vi "calculateDateFormate.vi"(8 "Error In":errorcluster, 11 "Shift":string) -> (0 "Error Out":errorcluster, 2 "Special Date Formate":string, 3 "Production Date":string)   [LabVIEW 2018]
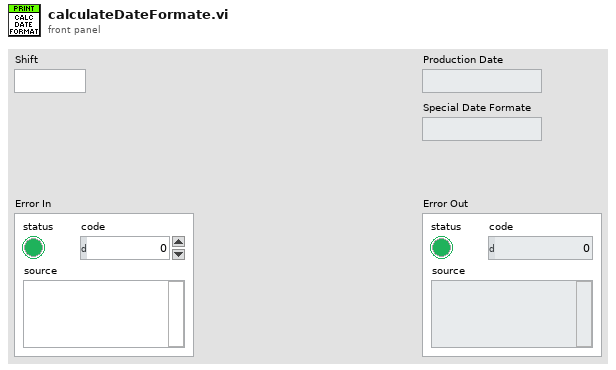
[diagram p1: front panel]
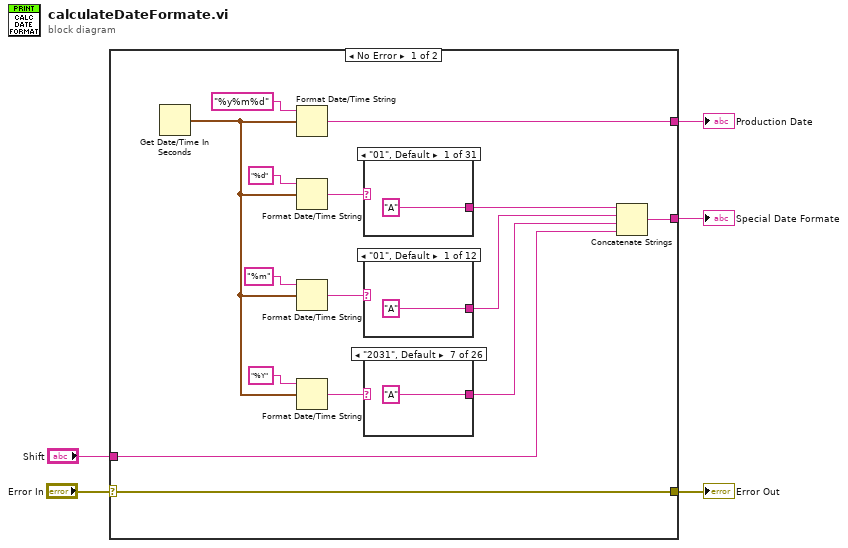
[diagram p0: block diagram]
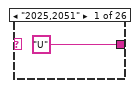
[diagram p2: hidden frame]
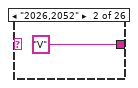
[diagram p3: hidden frame]
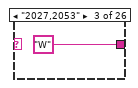
[diagram p4: hidden frame]
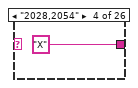
[diagram p5: hidden frame]
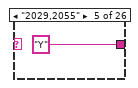
[diagram p6: hidden frame]
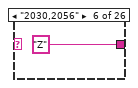
[diagram p7: hidden frame]
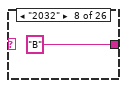
[diagram p8: hidden frame]
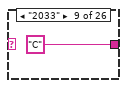
[diagram p9: hidden frame]
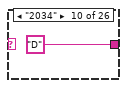
[diagram p10: hidden frame]
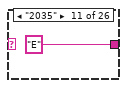
[diagram p11: hidden frame]
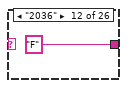
[diagram p12: hidden frame]
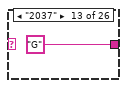
[diagram p13: hidden frame]
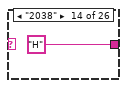
[diagram p14: hidden frame]
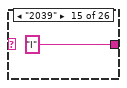
[diagram p15: hidden frame]
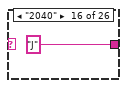
[diagram p16: hidden frame]
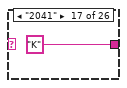
[diagram p17: hidden frame]
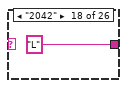
[diagram p18: hidden frame]
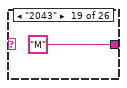
[diagram p19: hidden frame]
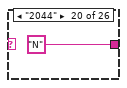
[diagram p20: hidden frame]
diagram:
  n1 = case shown="No Error" "Error In" {
    selector: "Error In" -> [w20 w90]
    tunnel: [w20 w90] -> w4
    tunnel: "Shift" -> [w10 _]
    tunnel: [w9 _] -> w2
    tunnel: [w6 _] -> w1
    frame No Error {
      n2 = Get Date/Time In Seconds() -> (seconds since 1Jan1904=w7:timestamp)
      n3 = Format Date/Time String(time format string (%c)="%y%m%d", seconds (now)=w7) -> (date/time string=w6:string)  [unwired: 1 in]
      n4 = Format Date/Time String(time format string (%c)="%d", seconds (now)=w7) -> (date/time string=w17:string)  [unwired: 1 in]
      n5 = Format Date/Time String(time format string (%c)="%m", seconds (now)=w7) -> (date/time string=w18:string)  [unwired: 1 in]
      n6 = Format Date/Time String(time format string (%c)="%Y", seconds (now)=w7) -> (date/time string=w19:string)  [unwired: 1 in]
      n7 = case shown="\"01\", Default" w17 {
        tunnel: ["A" "B" "C" "D" "E" "F" "G" "H" "I" "J" "K" "L" "M" "N" "O" "P" "Q" "R" "S" "T" "U" "V" "W" "X" "Y" "Z" "1" "2" "3" "4" "5"] -> w13
        frame "01", Default {
        }
        frame "02" {
        }
        frame "03" {
        }
        frame "04" {
        }
        frame "05" {
        }
        frame "06" {
        }
        frame "07" {
        }
        frame "08" {
        }
        frame "09" {
        }
        frame "10" {
        }
        frame "11" {
        }
        frame "12" {
        }
        frame "13" {
        }
        frame "14" {
        }
        frame "15" {
        }
        frame "16" {
        }
        frame "17" {
        }
        frame "18" {
        }
        frame "19" {
        }
        frame "20" {
        }
        frame "21" {
        }
        frame "22" {
        }
        frame "23" {
        }
        frame "24" {
        }
        frame "25" {
        }
        frame "26" {
        }
        frame "27" {
        }
        frame "28" {
        }
        frame "29" {
        }
        frame "30" {
        }
        frame "31" {
        }
      }
      n8 = case shown="\"01\", Default" w18 {
        tunnel: ["A" "B" "C" "D" "E" "F" "G" "H" "I" "J" "K" "L"] -> w12
        frame "01", Default {
        }
        frame "02" {
        }
        frame "03" {
        }
        frame "04" {
        }
        frame "05" {
        }
        frame "06" {
        }
        frame "07" {
        }
        frame "08" {
        }
        frame "09" {
        }
        frame "10" {
        }
        frame "11" {
        }
        frame "12" {
        }
      }
      n9 = case shown="\"2031\", Default" w19 {
        tunnel: ["U" "V" "W" "X" "Y" "Z" "A" "B" "C" "D" "E" "F" "G" "H" "I" "J" "K" "L" "M" "N" "O" "P" "Q" "R" "S" "T"] -> w11
        frame "2025,2051" {
        }
        frame "2026,2052" {
        }
        frame "2027,2053" {
        }
        frame "2028,2054" {
        }
        frame "2029,2055" {
        }
        frame "2030,2056" {
        }
        frame "2031", Default {
        }
        frame "2032" {
        }
        frame "2033" {
        }
        frame "2034" {
        }
        frame "2035" {
        }
        frame "2036" {
        }
        frame "2037" {
        }
        frame "2038" {
        }
        frame "2039" {
        }
        frame "2040" {
        }
        frame "2041" {
        }
        frame "2042" {
        }
        frame "2043" {
        }
        frame "2044" {
        }
        frame "2045" {
        }
        frame "2046" {
        }
        frame "2047" {
        }
        frame "2048" {
        }
        frame "2049" {
        }
        frame "2050" {
        }
      }
      n10 = Concatenate Strings(w13, w12, w11, w10) -> (w9:string)
    }
    frame Error {
    }
  }
  "Special Date Formate" <- w2
  "Error Out" <- w4
  "Production Date" <- w1
